vi "CVT2IndexWriteTest.vi"() -> (3 "Unit Test Framework Results":T1)   [LabVIEW 2013, in "UnitTests.lvlib"]
uses:
  UnitTests.lvlib
  <vilib>/utf/common/utf_test_result_troll.ctl
  <vilib>/utf/common/utf_test_result.ctl
  <vilib>/utf/common/utf_test_result_failure.ctl
  <vilib>/utf/common/utf_test_comparison_operators.ctl
  <vilib>/utf/common/utf_vi_tag.ctl
  <vilib>/NI/Current Value Table/DataTypes/I32_Write Index.vi
  <vilib>/NI/Current Value Table/DataTypes/I32_Read Index.vi
  <vilib>/NI/Current Value Table/Memory Block.vi
  <vilib>/NI/Current Value Table/DataTypes/I32_Memory Block.vi
  <vilib>/utf/NI_UnitTestFramework.lvlib
  <vilib>/NI/Current Value Table/Current Value Table.lvlib
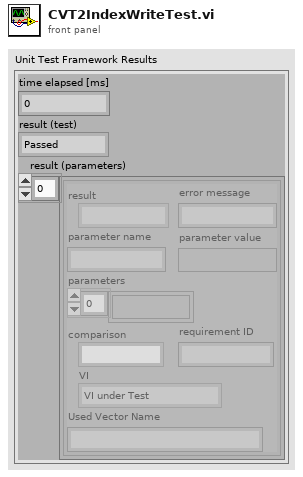
[diagram p1: front panel]
types:
  T1 = typedef "NI_UnitTestFramework.lvlib/utf_test_result_troll.ctl" = cluster{"time elapsed [ms]":u32, "result (test)":T2, "result (parameters)":T3[]}
  T2 = typedef "NI_UnitTestFramework.lvlib/utf_test_result.ctl" = enum16{"Passed", "Failed", "Error", "Skipped", "Not Processed"}
  T3 = typedef "NI_UnitTestFramework.lvlib/utf_test_result_failure.ctl" = cluster{"result":T2, "error message":string, "parameter name":string, "parameter value":variant, "parameters":variant[], "comparison":T4, "requirement ID":string, "VI":T5, "Used Vector Name":string}
  T4 = typedef "NI_UnitTestFramework.lvlib/utf_test_comparison_operators.ctl" = enum16{"=", "!=", ">", ">=", "<", "<=", "range", "symmetric tolerance", "asymmetric tolerance", "string contains", "string not contain", "array size", "string length", "array range", "by element", "array range (limit array)", "user-defined", "array contains", "array not contain", "vector length", "= (elm)", "!= (elm)", "= (case insensitive)", "!= (case insensitive)"}
  T5 = typedef "NI_UnitTestFramework.lvlib/utf_vi_tag.ctl" = enum16{"Setup VI", "VI under Test", "Teardown VI"}
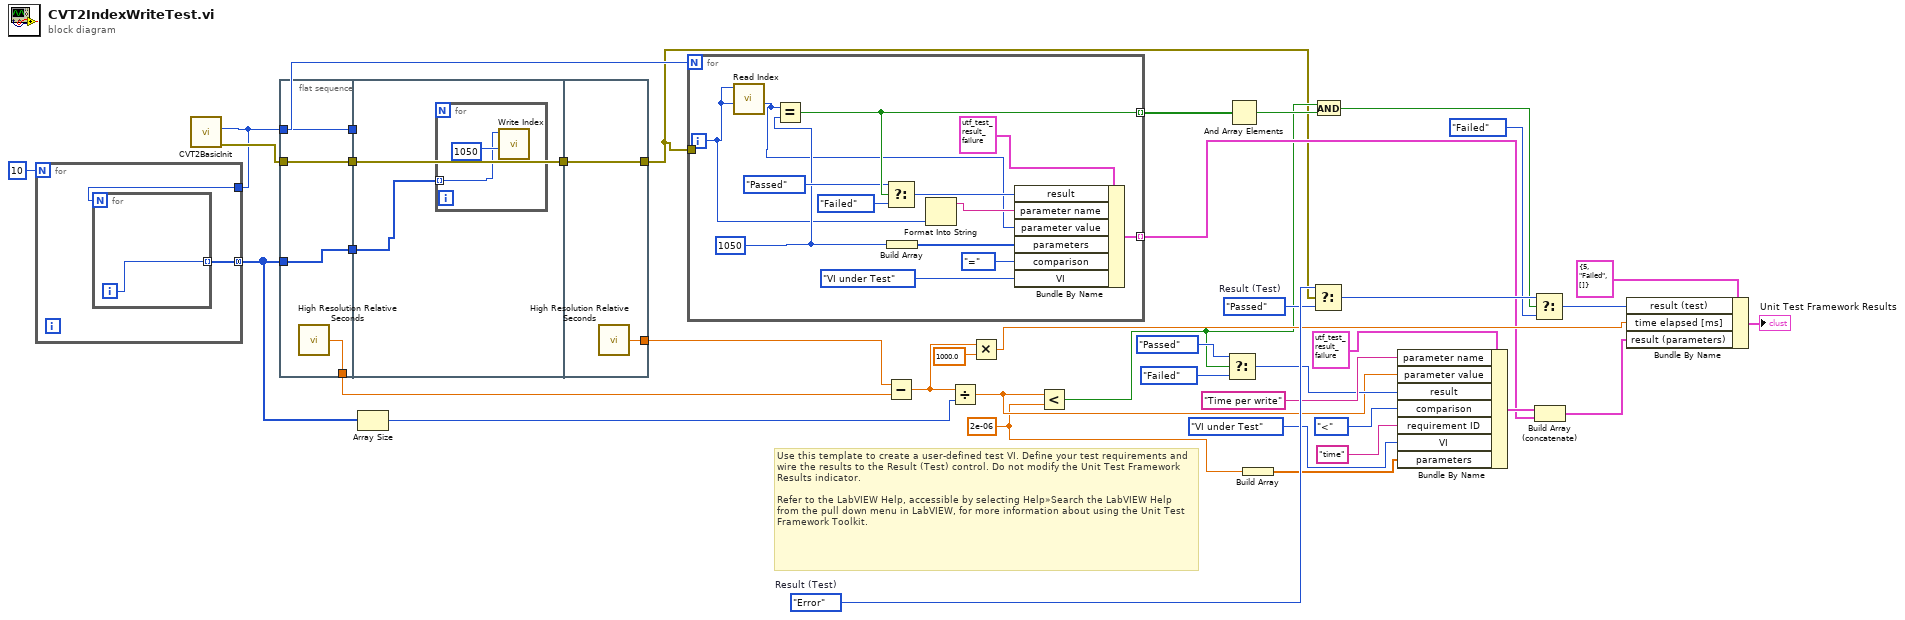
[diagram p0: block diagram]
diagram:
  w13 = 2e-06 ("y")
  w35 = utf_test_result."Error"  # Result (Test)
  w34 = utf_test_result."Passed"  # Result (Test)
  # "Use this template to create a user-defined test VI. Define your test requirements and wire the results to the Result (Test) control. Do not modify the Unit Test Framework Results indicator. \n\nRefer to the LabVIEW Help, accessible by selecting Help»Search the LabVIEW Help from the pull down menu in LabVIEW, for more information about using the Unit Test Framework Toolkit."
  n1 = call "CVT2BasicInit.vi"() -> ("error out"=w8:errorcluster, "Tags per type out"=w6:i32)  [unwired: 9 in, 1 out]
  n2 = for {
    N: 10 -> [_]
    tunnel: w6 -> [w42]
    tunnel: [w41] -> w3 mode=concatenating
    n3 = for {
      N: w42 -> [_]
      tunnel: [w43] -> w41 mode=indexing
      i -> [w43]
    }
  }
  n4 = flat-sequence {
    tunnel: [w47] -> w37
    tunnel: w8 -> [w45]
    tunnel: [w46] -> w29
    tunnel: w6 -> [w46]
    tunnel: [w45] -> w28
    tunnel: [w44] -> w4
    tunnel: w3 -> [w44]
    tunnel: w29 -> [_]
    tunnel: w28 -> [w49]
    tunnel: [w49] -> w7
    tunnel: w4 -> [w48]
    tunnel: [w53] -> w38
    tunnel: [w52] -> w1
    tunnel: w7 -> [w52]
    frame #0 {
      n5 = call <vilib>:"High Resolution Relative Seconds.vi"() -> ("relative seconds"=w47:dbl)
    }
    frame #1 {
      n6 = for {
        tunnel: w48 -> [w50] mode=indexing
        n7 = call-poly <vilib>:"Write Index.vi"("Value"=1050, "Index"=w50) -> ()  [unwired: 10 in]
      }
    }
    frame #2 {
      n8 = call <vilib>:"High Resolution Relative Seconds.vi"() -> ("relative seconds"=w53:dbl)
    }
  }
  n9 = Array Size(array=w3) -> (size(s)=w2:i32)
  n10 = for {
    N: w6 -> [_]
    tunnel: [w64] -> w25 mode=indexing
    tunnel: [w60] -> w11 mode=indexing
    tunnel: w1 -> [_]
    i -> [w55]
    w57 = 1050 ("Value")
    n11 = call-poly <vilib>:"Read Index.vi"("Default"=w55, "Index"=w55) -> ("Value"=w54:i32)  [unwired: 9 in]
    n12 = Equal?(x=w54, y=w57) -> (x = y?=w64:bool)
    n13 = Select(t=utf_test_result."Passed" ("result"), s=w64, f=utf_test_result."Failed" ("result")) -> (s? t:f=w61:T2)
    n14 = Build Array(w57) -> (w58:i32[])
    n15 = Format Into String(w55) -> (resulting string=w56:string)  [unwired: 3 in, 1 out]
    n16 = Bundle By Name(cluster=T3 {"result"=enum."Passed", "error message"="", "parameter name"="", "parameter value"=variant, "parameters"=[], "comparison"=enum."=", "requirement ID"="", "VI"=enum."Setup VI", "Used Vector Name"=""} ("Unit Test Framework - result (parameters)"), "result"=w61, "parameter name"=w56, "parameter value"=w54, "parameters"=w58, "comparison"=utf_test_comparison_operators."=", "VI"=utf_vi_tag."VI under Test") -> (w60:T3)
  }
  n17 = Subtract(x=w38, y=w37) -> (x-y=w27:dbl)
  n18 = Divide(x=w27, y=w2) -> (x/y=w16:dbl)
  n19 = Multiply(x=w27, y=1000.0) -> (x*y=w30:dbl)
  n20 = Less?(x=w16, y=w13) -> (x < y?=w9:bool)
  n21 = Select(t=utf_test_result."Passed" ("result"), s=w9, f=utf_test_result."Failed" ("result")) -> (s? t:f=w17:T2)
  n22 = And Array Elements(Boolean array=w25) -> (logical AND=w24:bool)
  n23 = Build Array(w13) -> (w12:dbl[])
  n24 = Select(t=w35, s=w1, f=w34) -> (s? t:f=w23:T2)
  n25 = And(x=w9, y=w24) -> (x .and. y?=w10:bool)
  n26 = Bundle By Name(cluster=T3 {"result"=enum."Passed", "error message"="", "parameter name"="", "parameter value"=variant, "parameters"=[], "comparison"=enum."=", "requirement ID"="", "VI"=enum."Setup VI", "Used Vector Name"=""} ("Unit Test Framework - result (parameters)"), "parameter name"="Time per write", "parameter value"=w16, "result"=w17, "comparison"=utf_test_comparison_operators."<", "requirement ID"="time", "VI"=utf_vi_tag."VI under Test", "parameters"=w12) -> (w33:T3)
  n27 = Select(t=w23, s=w10, f=utf_test_result."Failed") -> (s? t:f=w21:T2)
  n28 = Build Array (concatenate)(w33, w11) -> (w32:T3[])
  n29 = Bundle By Name(cluster=T1 {"time elapsed [ms]"=5, "result (test)"=enum."Failed", "result (parameters)"=[]} ("Unit Test Framework - Result"), "result (test)"=w21, "time elapsed [ms]"=w30, "result (parameters)"=w32) -> (→"Unit Test Framework Results":T1)
